vi "setCol4ColorAccordingToChkResult.vi"(8 "error in":errorcluster, 9 "rowNum":i32, 10 "judgeRes":string, 11 "Tbl Refnum in":refnum<vi>) -> (0 "error out":errorcluster, 3 "Tbl Refnum Out":refnum<vi>)   [LabVIEW 2010]
uses:
  <vilib>/Utility/miscctls.llb/LVRowAndColumnTypeDef.ctl
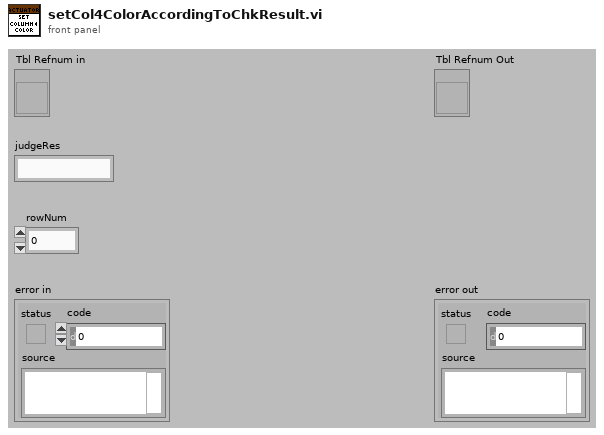
[diagram p1: front panel]
types:
  T1 = typedef "LVRowAndColumnTypeDef.ctl" = cluster{"Row":i32, "Column":i32}
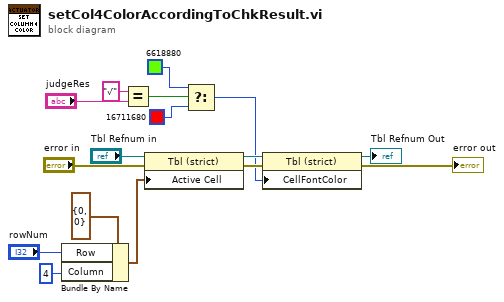
[diagram p0: block diagram]
diagram:
  n1 = Bundle By Name(cluster=T1 {"Row"=0, "Column"=0} ("Active Cell:Active Cell"), "Row"="rowNum", "Column"=4) -> (w10:T1)
  n2 = Equal?(x="√", y="judgeRes") -> (x = y?=w13:bool)
  n3 = property on="Property Node" class="Tbl (strict)"(reference="Tbl Refnum in", error in="error in", "Active Cell"=w10) -> (reference out=w9:refnum<vi>, error out=w8:errorcluster)
  n4 = Select(t=u32 6618880, s=w13, f=u32 16711680) -> (s? t:f=w7:u32)
  n5 = property on="Property Node" class="Tbl (strict)"(reference=w9, error in=w8, "CellFontColor"=w7) -> (reference out=→"Tbl Refnum Out":refnum<vi>, error out=→"error out":errorcluster)
